vi "Resolve-client-type.vi"(8 "error in (no error)":errorcluster, 10 "Module name":string, 11 "ModComm in":T2) -> (0 "error out":errorcluster, 1 "Supported?":bool, 2 "Module type":T1, 3 "ModComm out":T2)   [LabVIEW 2013, in "Server.lvlib" / "Server.lvclass"]
uses:
  Server.lvclass
  Object-reference.ctl
  Supported-module-types.ctl
  Custom-errors.ctl
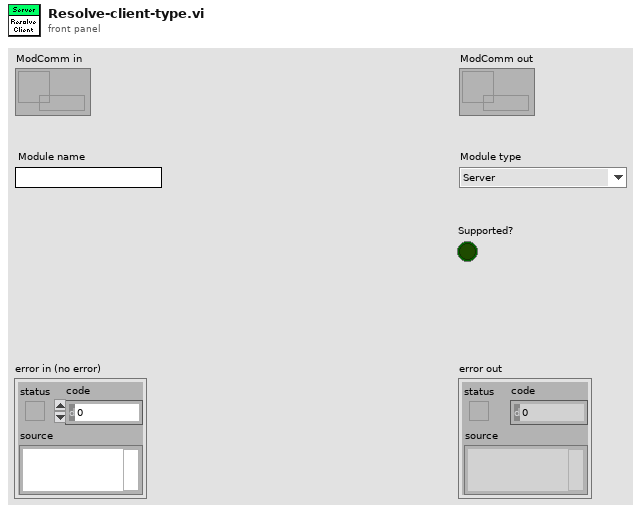
[diagram p1: front panel]
types:
  T1 = typedef "Server.lvlib/Server.lvclass/Supported-module-types.ctl" = enum16{"Server", "All", "BeamControl", "PowderDeposition", "StrategyParser", "CameraVision", "MaterialCharacterization", "StatusMonitor", "SLMSimulation", "LaserCharacterization"}
  T2 = typedef "Server.lvlib/Server.lvclass/Object-reference.ctl" = refnum<data-value>
  T3 = typedef "Server.lvlib/Server.lvclass/Custom-errors.ctl" = enum16{"Not implemented", "Command not recognized", "Invalid input", "Timeout", "Client not allowed", "Max clients reached"}
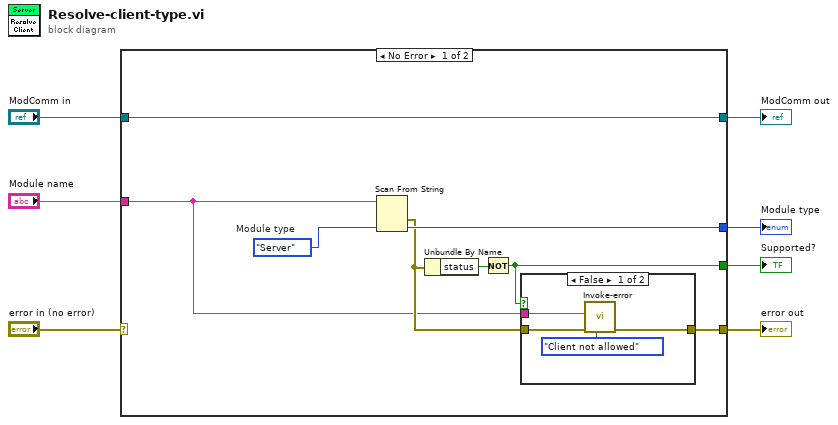
[diagram p0: block diagram]
diagram:
  n1 = case shown="No Error" "error in (no error)" {
    selector: "error in (no error)" -> [_ w22]
    tunnel: [w10 w22] -> w6
    tunnel: [w15 w21] -> w4
    tunnel: "ModComm in" -> [w15 w21]
    tunnel: "Module name" -> [w9 _]
    tunnel: [w13 _] -> w2
    tunnel: [w8 _] -> w1
    frame No Error {
      w14 = Supported-module-types."Server"  # Module type
      n2 = Scan From String(input string=w9, default 1=w14) -> (error out=w11:errorcluster, output 1=w13:T1)  [unwired: 3 in, 2 out]
      n3 = Unbundle By Name(w11) -> ("status"=w12:bool)
      n4 = Not(x=w12) -> (.not. x?=w8:bool)
      n5 = case shown="False" w8 {
        tunnel: w11 -> [w19 w20]
        tunnel: [w18 w20] -> w10
        tunnel: w9 -> [w16 _]
        frame False {
          n6 = call "Invoke-error.vi"("Error"=Custom-errors."Client not allowed", "error in (no error)"=w19, "Additional message"=w16) -> ("error out"=w18:errorcluster)  [unwired: 8 in]
        }
        frame True {
        }
      }
    }
    frame Error {
    }
  }
  "error out" <- w6
  "ModComm out" <- w4
  "Supported?" <- w1
  "Module type" <- w2
